vi "FTT Sreen.vi"(8 "error in (no error)":errorcluster caption="错误输入（无错误）", 11 "Main":T2={"Tite"="", "Base path"=path "", "Table"=[], "Stations"=[], "Shield Array"=[], "UPHs"=[], "VISA"={"VISA"="", "baud rate"=9600, "data bits"=8, "parity"=enum."None", "stop bits"=10, "flow control"=0}, "Path"={"roof"=path "", "Config"=path "", "Png"=path ""}, "Ctr"={"DB Dispaly"=refnum, "Error Table"=refnum, "Display"=refnum, "Login"=refnum, "Exit"=refnum, "FTT_Submit"=refnum}, "Login"={"User"="", "Grade"=""}, "information"={"cause"="", "Type"=enum."Inform", "code"=0, "Suroce"="", "Status"=FALSE}, "Local DB"={"Connstr"="", "Database"={"Constr"={"Driver"="", "Server"="", "User"="", "Pwd"="", "Database"=""}, "conn ref"=refnum, "State"=FALSE}}, "Remote DB"={"Connstr"="", "Database"={"Constr"={"Driver"="", "Server"="", "User"="", "Pwd"="", "Database"=""}, "conn ref"=refnum, "State"=FALSE}}, "FTT TV"="", "ExchangeTime"=0, "NVH"="", "EOL Path"=path ""} {"VISA"."flow control" items=["None", "XON/XOFF", "RTS/CTS", "XON/XOFF & RTS/CTS", "DTR/DSR", "XON/XOFF & DTR/DSR"]; "VISA"."stop bits" items=["1.0"=10, "1.5"=15, "2.0"=20]}) -> (0 "error out":errorcluster)   [LabVIEW 2014]
uses:
  Type'def/CN Product1_5 Ctr.ctl
  Type'def/CN Product1_4 Ctr.ctl
  Type'def/CN Product Ctr.ctl
  Type'def/Tab.ctl
  Type'def/MainCtr.ctl
  Type'def/UPH Config.ctl
  SubVI's/VISA/Ctr/VISA Ctr.ctl
  Type'def/Main Ctr Ref.ctl
  Type'def/User Login.ctl
  SubVI's/Database/Ctr/Conneect State.ctl
  SubVI's/Database/Ctr/Constr.ctl
  <vilib>/addons/database/Connection.llb/Conn ObjectReference.ctl
  Type'def/CN image Ctr.ctl
  <vilib>/picture/picture.llb/imagedata.ctl
  Type'def/CN Config Ctr.ctl
  <vilib>/addons/database/NI_Database_API.lvlib
panel:
  out "Tab":T1(array[ring])
  out "size(s)":i32
  out "Value":string
  out "Repaired":string
  out "Slash 04":string
  out "End?":bool
  out "Show Tab":T10
  out "Tab CN":enum32{"1/2", "1/3", "1/4", "1/5", "2/5", "3/5"}(tab)
  out "CN image2/2":T11
  out "CN image1/2":T11
  out "CN image3/3":T11
  out "CN image2/3":T11
  out "CN image1/3":T11
  out "CN image4/4":T12
  out "CN image3/4":T12
  out "CN image2/4":T12
  out "CN image1/4":T12
  out "CN image5/5":T13
  out "CN image4/5":T13
  out "CN image3/5":T13
  out "CN image2/5":T13
  out "CN image1/5":T13
  out "CN image5/6":T13
  out "CN image4/6":T13
  out "CN image3/6":T13
  out "CN image2/6":T13
  out "CN image1/6":T13
  out "CN image5/7":T13
  out "CN image4/7":T13
  out "CN image3/7":T13
  out "CN image2/7":T13
  out "CN image1/7":T13
  out "Roof Picture":picture
  out "Vehicle Picture":picture
  out "Line status":string
  out "UPH status":string
  out "Rollo Color status":string
  out "Model":string
  out "Slash 03":string
  out "Slash 01":string
  out "Slash 02":string
  out "FTT Rate":string
  out "Reject":string
  out "Target(%)":string
  out "Target now":string
  out "FTT":string
  out "Actual":string
  out "Plan":string
  out "Repaired and Reject Title":string
  out "Target and Actual Title":string
  out "FTT and FTT Rate Title":string
  out "Plan and Rate Title":string
  out "Error Info 3":string
  out "Error Info 2":string
  out "Error Info":string
  out "Error BG":u32(colorbox)
  out "Time":string
  out "Date":string
  out "Title":string
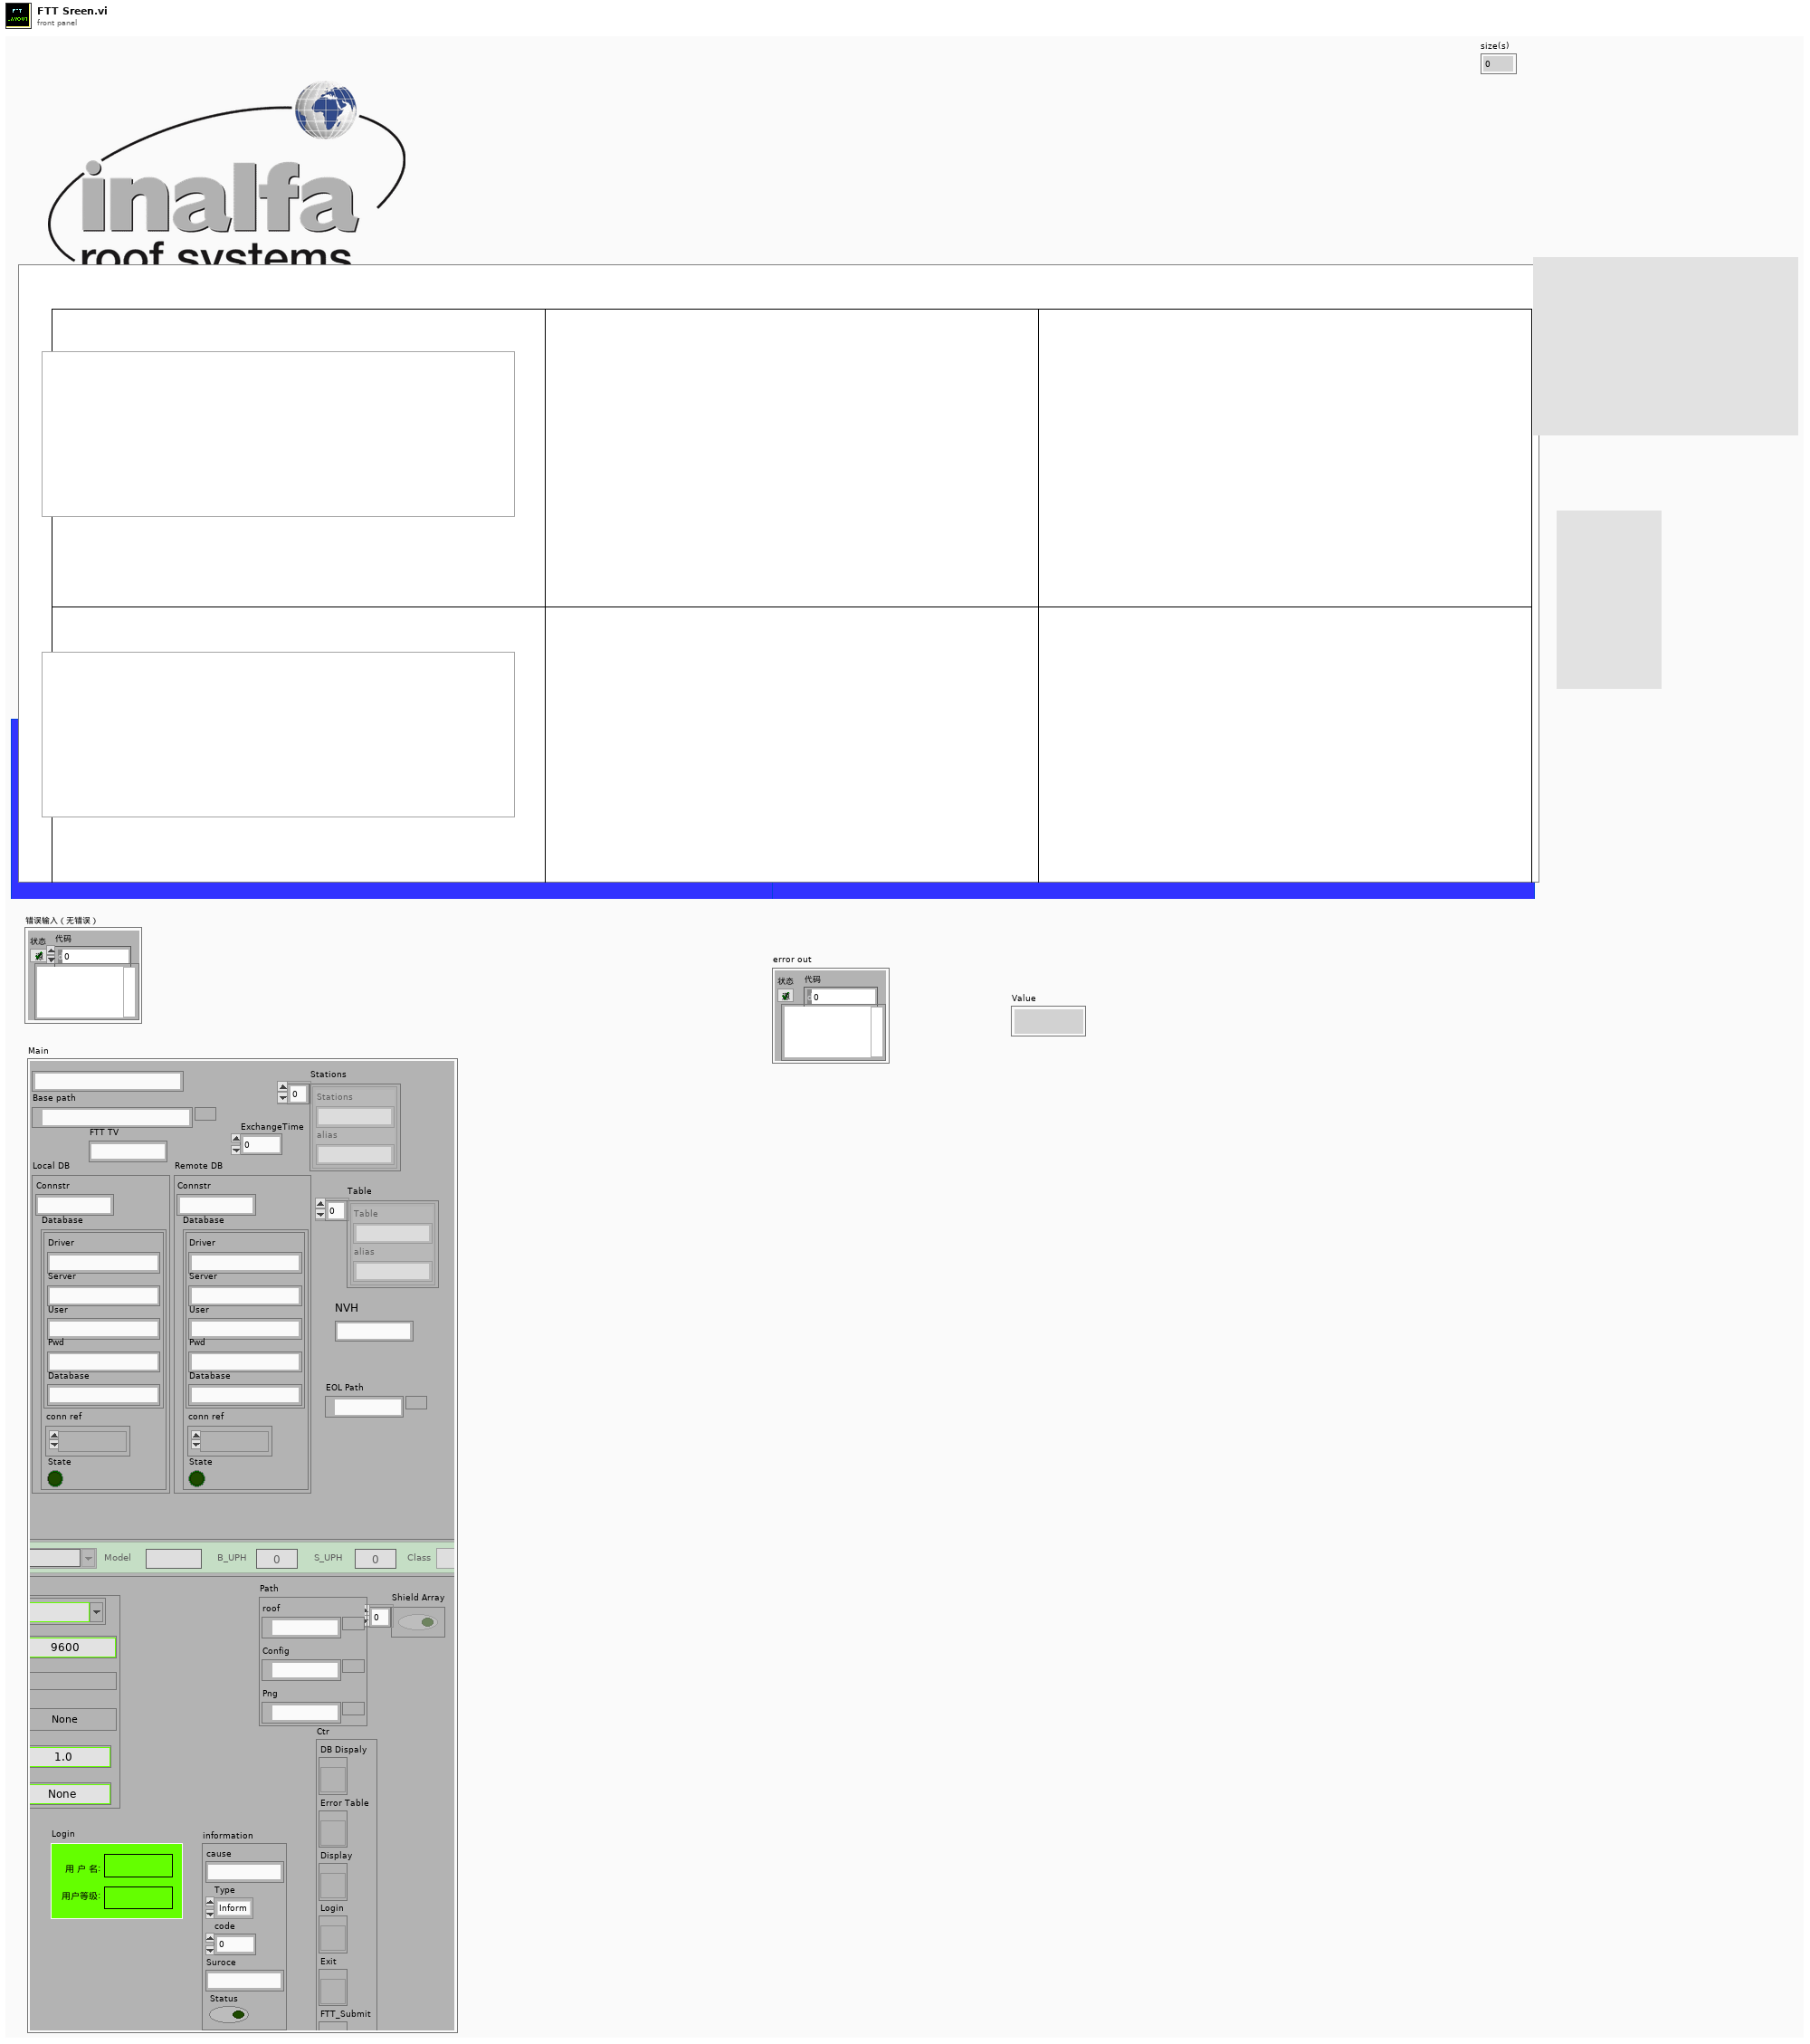
[diagram p1: front panel]
types:
  T1 = enum32{"1/2", "1/3", "1/4", "1/5", "2/5", "3/5"}[]
  T2 = typedef "MainCtr.ctl" = cluster{"Tite":string, "Base path":path, "Table":cluster{"Table":string, "alias":string}[], "Stations":cluster{"Stations":string, "alias":string}[], "Shield Array":bool[], "UPHs":T3[], "VISA":T4, "Path":cluster{"roof":path, "Config":path, "Png":path}, "Ctr":T5, "Login":T6, "information":cluster{"cause":string, "Type":enum16{"Inform", "Warning", "Alarm"}, "code":i32, "Suroce":string, "Status":bool}, "Local DB":cluster{"Connstr":string, "Database":T7}, "Remote DB":cluster{"Connstr":string, "Database":T7}, "FTT TV":string, "ExchangeTime":i32, "NVH":string, "EOL Path":path}
  T3 = typedef "UPH Config.ctl" = cluster{"Line_No":string, "Model":string, "B_UPH ":i16, "S_UPH  ":i16, "Class":enum16{"Big", "Small"}}
  T4 = typedef "VISA Ctr.ctl" = cluster{"VISA":refnum<visa-resource-name>, "baud rate":u32, "data bits":u16, "parity":enum16{"None", "Odd", "Even", "Mark", "Space"}, "stop bits":u16, "flow control":u16}
  T5 = typedef "Main Ctr Ref.ctl" = cluster{"DB Dispaly":refnum<vi>, "Error Table":refnum<vi>, "Display":refnum<vi>, "Login":refnum<vi>, "Exit":refnum<vi>, "FTT_Submit":refnum<vi>}
  T6 = typedef "User Login.ctl" = cluster{"User":string, "Grade":string}
  T7 = typedef "Conneect State.ctl" = cluster{"Constr":T8, "conn ref":T9, "State":bool}
  T8 = typedef "Constr.ctl" = cluster{"Driver":string, "Server":string, "User":string, "Pwd":string, "Database":string}
  T9 = typedef "NI_Database_API.lvlib/Conn ObjectReference.ctl" = refnum<k1>
  T10 = typedef "Tab.ctl" = enum32{"Customer and Shift Info", "Manufacture Info", "Device error info"}
  T11 = typedef "CN Product Ctr.ctl" = cluster{"2D Picture 3":picture, "Model":string, "Brand":string}
  T12 = typedef "CN Product1_4 Ctr.ctl" = cluster{"2D Picture 3":picture, "Model":string, "Brand":string}
  T13 = typedef "CN Product1_5 Ctr.ctl" = cluster{"2D Picture 3":picture, "Model":string, "Brand":string}
  T14 = typedef "imagedata.ctl" = cluster{"image type":i32, "image depth":i32, "image":u8[], "mask":u8[], "colors":u32[], "Rectangle":cluster{"left":i16, "top":i16, "right":i16, "bottom":i16}}
  T15 = cluster{"FTTColor":cluster{"Low":u32, "Middle":u32, "High":u32}, "TargetColor":cluster{"Low":u32, "Middle":u32, "High":u32}}
  T16 = cluster{"FTTRate":cluster{"Low":u32, "High":u32}, "TargetRate":cluster{"Low":u32, "High":u32}}
  T17 = typedef "CN image Ctr.ctl" = cluster{"Images":T14[], "filenames":string[], "Fit Zoom":dbl[], "CN Config":T18[], "CN Enable":T18[], "image Enable":T14[], "CN Ref Enable":refnum<vi>[], "Tab ":enum32{"1/2", "1/3", "1/4", "1/5", "2/5", "3/5"}[], "Pic Enable":refnum<vi>[]}
  T18 = typedef "CN Config Ctr.ctl" = cluster{"Model":string, "Pic_Name":string, "CarName":string, "En/Disable":bool}
  T19 = cluster{"Path":cluster{"roof":path, "Config":path, "Png":path}, "Exit":refnum<vi>, "Show Tab":refnum<vi>, "Target(%)":refnum<vi>, "Repaired":refnum<vi>, "Reject":refnum<vi>, "FTT":refnum<vi>, "FTT Rate":refnum<vi>, "Line status":refnum<vi>, "Vehicle Picture":refnum<vi>, "Roof Picture":refnum<vi>, "Time":refnum<vi>, "Date":refnum<vi>, "Title":refnum<vi>, "Error Info":refnum<vi>, "UPH status":refnum<vi>, "Rollo Color status":refnum<vi>, "Plan":refnum<vi>, "Actual":refnum<vi>, "Repaired":refnum<vi>, "Target now":refnum<vi>, "Range":cluster{"FTTRate":cluster{"Low":u32, "High":u32}, "TargetRate":cluster{"Low":u32, "High":u32}}, "Color":cluster{"FTTColor":cluster{"Low":u32, "Middle":u32, "High":u32}, "TargetColor":cluster{"Low":u32, "Middle":u32, "High":u32}}, "Ctr Color":cluster{"Label":string, "Color":u32}[], "CN Ctr Ref":refnum<vi>[], "CN image":T17, "Tab CN":refnum<vi>}
  T20 = cluster{"seconds":dbl, "Pages":i32, "element":enum32{"1/2", "1/3", "1/4", "1/5", "2/5", "3/5"}}
  T21 = typedef "Main FTT.ctl" = cluster{"Line_Name":string, "Model":string, "Line_State":string, "Color":string, "UPH":string, "Plan":string, "Target Rate":string, "Target":string, "Actual":string, "FTT":string, "FTT Rate":string, "Repaired":string, "Reject":string}
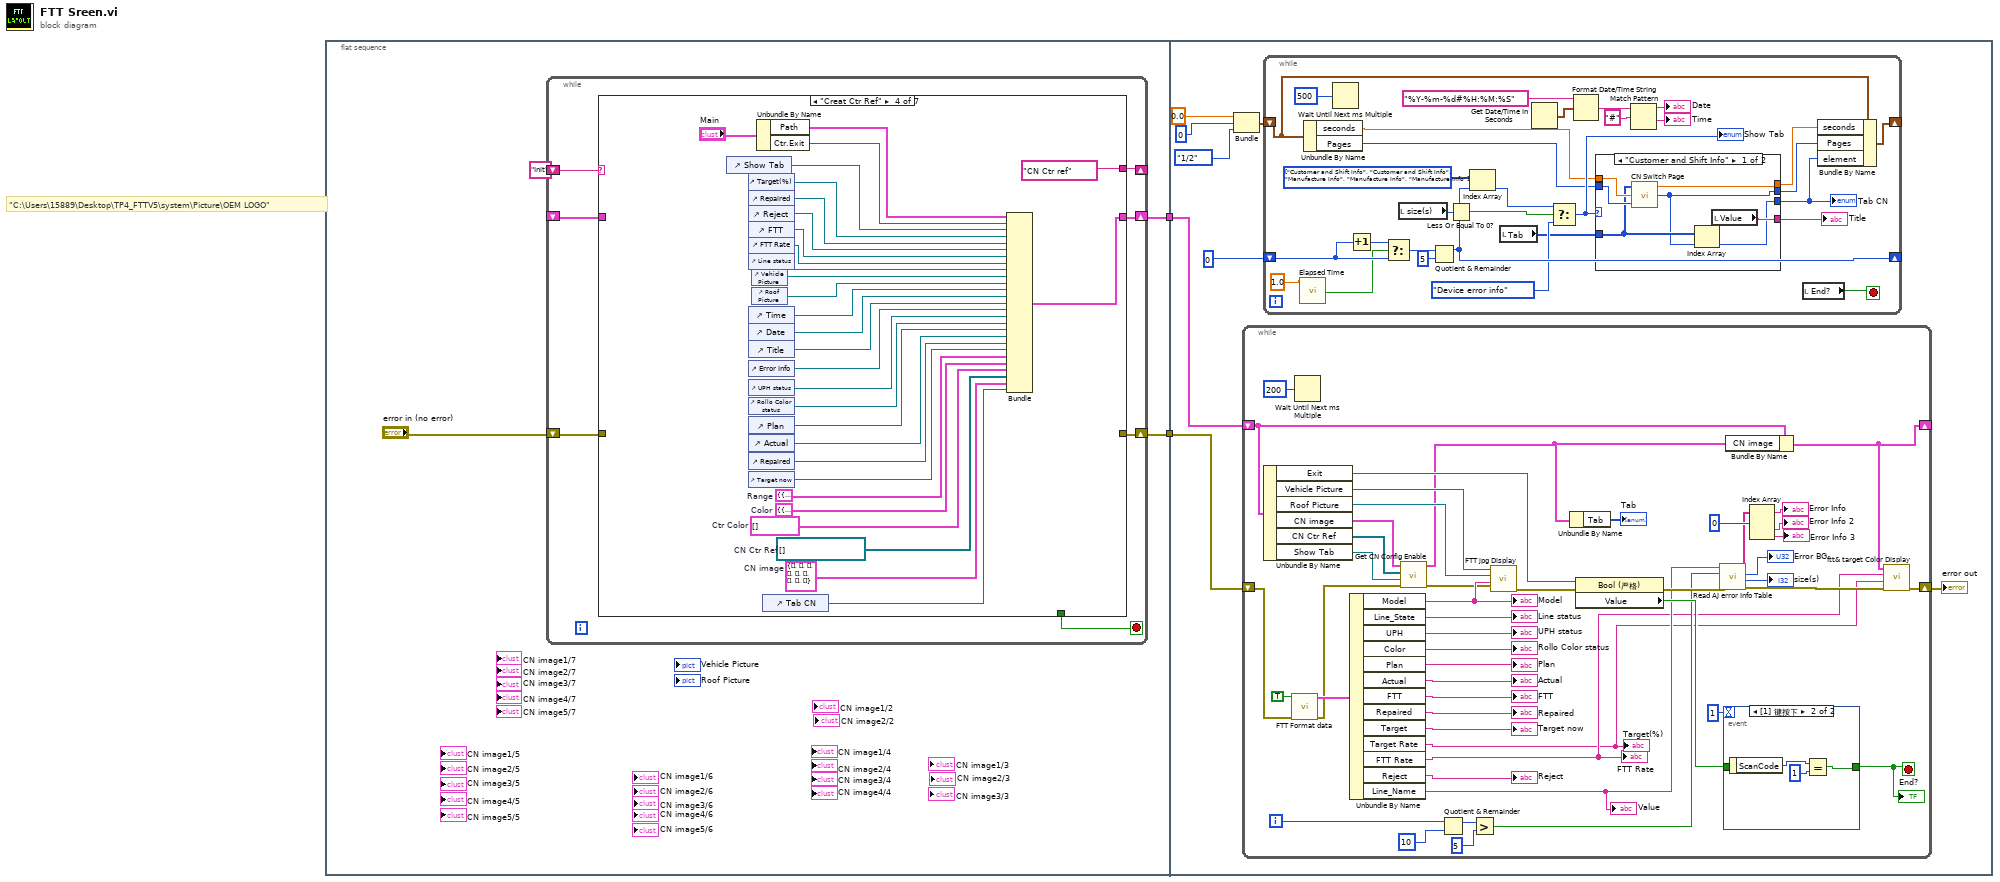
[diagram p0: block diagram]
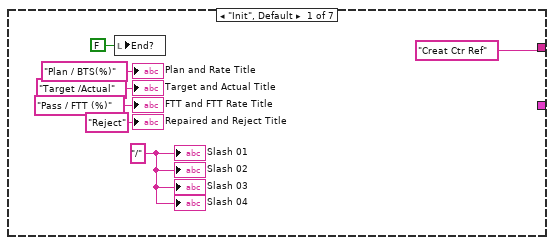
[diagram p2: hidden frame]
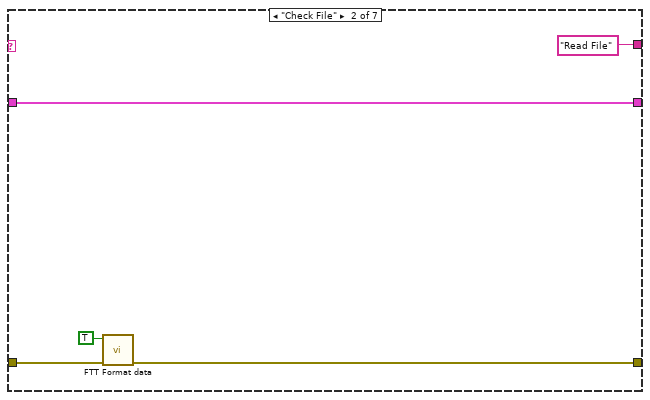
[diagram p3: hidden frame]
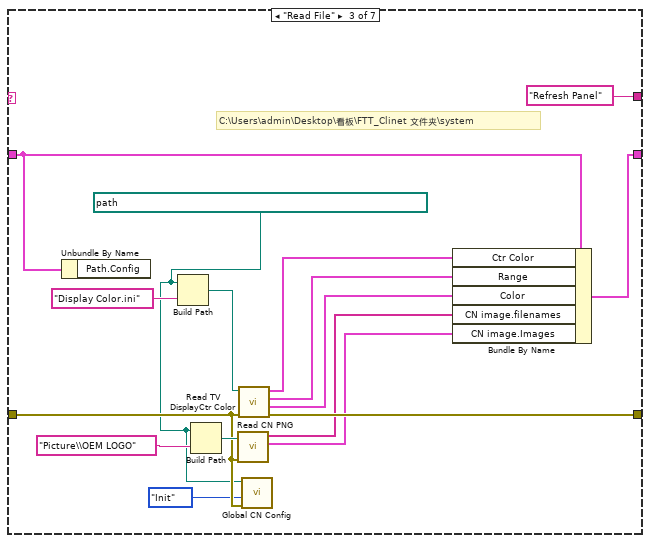
[diagram p4: hidden frame]
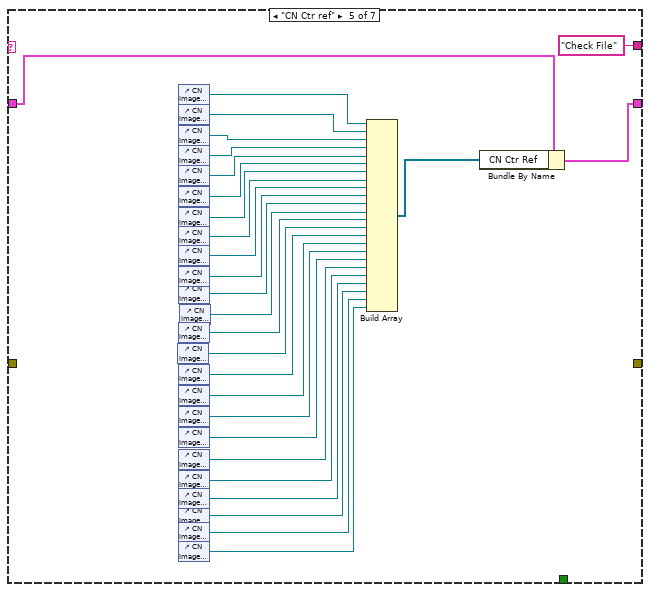
[diagram p5: hidden frame]
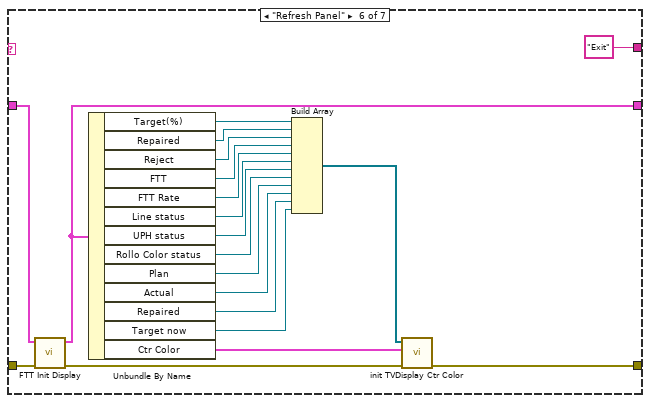
[diagram p6: hidden frame]
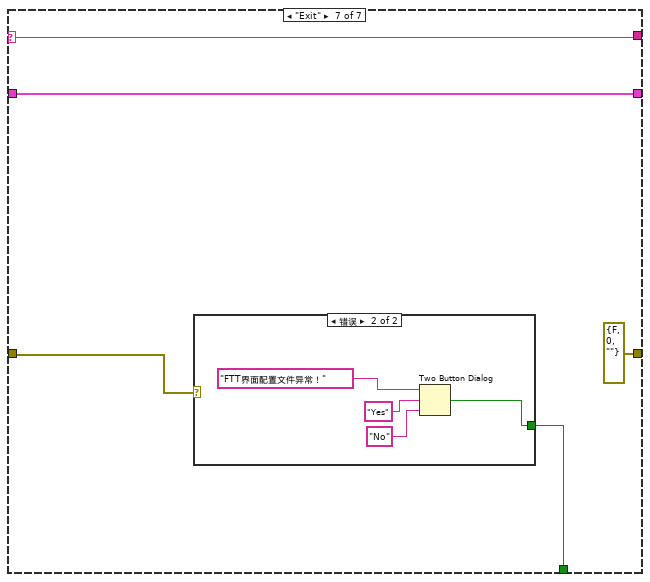
[diagram p7: hidden frame]
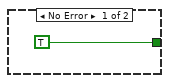
[diagram p8: hidden frame]
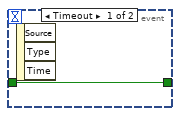
[diagram p9: hidden frame]
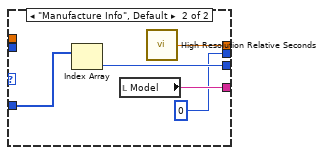
[diagram p10: hidden frame]
diagram:
  # "\"C:\\Users\\15889\\Desktop\\TP4_FTTV5\\system\\Picture\\OEM LOGO\""
  n1 = flat-sequence {
    tunnel: [w4] -> w2
    tunnel: [w3] -> w1
    tunnel: w2 -> [w136]
    tunnel: w1 -> [w137]
    frame #0 {
      n2 = while {
        shift-right: [w12] -> _
        shift-left: "Init" -> [w13]
        shift-right: [w10] -> w3
        shift-left: _ -> [w9]
        shift-right: [w7] -> w4
        shift-left: "error in (no error)" -> [w8]
        stop <- w11 stop-if-true
        n3 = case shown="\"Creat Ctr Ref\"" w13 {
          selector: w13 -> [_ _ _ _ _ _ w123]
          tunnel: ["Creat Ctr Ref" "Read File" "Refresh Panel" "CN Ctr ref" "Check File" "Exit" w123] -> w12
          tunnel: [_ _ _ _ _ _ w120] -> w11
          tunnel: [_ w24 w36 w59 w98 w100 w124] -> w10
          tunnel: w9 -> [_ w24 w37 _ w99 w101 w124]
          tunnel: w8 -> [_ w23 w28 _ _ w118 w121]
          tunnel: [_ w22 w38 _ _ w102 errorcluster {"status"=FALSE, "code"=0, "source"=""} ("error out")] -> w7
          frame "Init", Default {
            w16 = "/" ("Slash 01")
            n4 = local write "End?"(FALSE ("End?")) -> ()
            "FTT and FTT Rate Title" <- "Pass / FTT (%)" ("FTT Title")
            "Plan and Rate Title" <- "Plan / BTS(%)" ("Target and Color Title")
            "Target and Actual Title" <- "Target /Actual" ("FTT Title 3")
            "Repaired and Reject Title" <- "Reject" ("FTT Title 4")
            "Slash 02" <- w16
            "Slash 01" <- w16
            "Slash 03" <- w16
            "Slash 04" <- w16
          }
          frame "Check File" {
            n5 = call "FTT Format data.vi"("error in (no error)"=w23, "W/R"=TRUE) -> ("error out"=w22:errorcluster)  [unwired: 7 in, 2 out]
          }
          frame "Read File" {
            w26 = path "C:/Users/admin/Desktop/看板/FTT_Clinet 文件夹/system" ("Path.Config")
            # "C:\\Users\\admin\\Desktop\\看板\\FTT_Clinet 文件夹\\system"
            n6 = Unbundle By Name(w37) -> ()  [unwired: 1 out]
            n7 = Build Path(base path=w26, name or relative path="Display Color.ini") -> (appended path=w39:path)
            n8 = Build Path(base path=w26, name or relative path="Picture\\OEM LOGO") -> (appended path=w32:path)
            n9 = call "Read CN PNG.vi"("error in (no error)"=w28, "floder Path"=w32) -> ("Images"=w29:T14[], "filenames"=w30:string[])  [unwired: 7 in, 1 out]
            n10 = call "Read TV DisplayCtr Color.vi"("error in (no error)"=w28, "Path"=w39) -> ("error out"=w38:errorcluster, "Color"=w33:T15, "Range"=w34:T16, "Array"=w35:cluster{"Label":string, "Color":u32}[])  [unwired: 6 in]
            n11 = call "Global CN Config.vi"("error in (no error)"=w28, "Mode"=enum16{"Init", "Read", "Write"}."Init", "Path"=w26) -> ()  [unwired: 7 in, 2 out]
            n12 = Bundle By Name(cluster=w37, "Ctr Color"=w35, "Range"=w34, "Color"=w33, "CN image.filenames"=w30, "CN image.Images"=w29) -> (w36:T19)
          }
          frame "Creat Ctr Ref" {
            w43 = T17 {"Images"=[], "filenames"=[], "Fit Zoom"=[], "CN Config"=[], "CN Enable"=[], "image Enable"=[], "CN Ref Enable"=[], "Tab "=[], "Pic Enable"=[]}  # CN image
            w44 = refnum<vi>[] []  # CN Ctr Ref
            w47 = cluster{"Label":string, "Color":u32}[] []  # Ctr Color
            w48 = T15 {"FTTColor"={"Low"=0, "Middle"=0, "High"=0}, "TargetColor"={"Low"=0, "Middle"=0, "High"=0}}  # Color
            w49 = T16 {"FTTRate"={"Low"=0, "High"=0}, "TargetRate"={"Low"=0, "High"=0}}  # Range
            n13 = control-ref of="Show Tab"() -> (w71:refnum<vi>)
            n14 = control-ref of="Target(%)"() -> (w70:refnum<vi>)
            n15 = control-ref of="Repaired"() -> (w69:refnum<vi>)
            n16 = control-ref of="Reject"() -> (w68:refnum<vi>)
            n17 = control-ref of="FTT"() -> (w67:refnum<vi>)
            n18 = control-ref of="FTT Rate"() -> (w66:refnum<vi>)
            n19 = control-ref of="Line status"() -> (w65:refnum<vi>)
            n20 = control-ref of="Time"() -> (w62:refnum<vi>)
            n21 = control-ref of="Date"() -> (w61:refnum<vi>)
            n22 = control-ref of="Title"() -> (w60:refnum<vi>)
            n23 = control-ref of="Error Info"() -> (w56:refnum<vi>)
            n24 = control-ref of="UPH status"() -> (w55:refnum<vi>)
            n25 = control-ref of="Rollo Color status"() -> (w54:refnum<vi>)
            n26 = control-ref of="Plan"() -> (w53:refnum<vi>)
            n27 = control-ref of="Actual"() -> (w52:refnum<vi>)
            n28 = control-ref of="Repaired"() -> (w51:refnum<vi>)
            n29 = control-ref of="Target now"() -> (w50:refnum<vi>)
            n30 = control-ref of="Vehicle Picture"() -> (w64:refnum<vi>)
            n31 = control-ref of="Roof Picture"() -> (w63:refnum<vi>)
            n32 = Unbundle By Name("Main") -> ("Path"=w45:cluster{"roof":path, "Config":path, "Png":path}, "Ctr.Exit"=w57:refnum<vi>)
            n33 = control-ref of="Tab CN"() -> (w42:refnum<vi>)
            n34 = Bundle("Path"=w45, "Exit"=w57, "Show Tab"=w71, "Target(%)"=w70, "Repaired"=w69, "Reject"=w68, "FTT"=w67, "FTT Rate"=w66, "Line status"=w65, "Vehicle Picture"=w64, "Roof Picture"=w63, "Time"=w62, "Date"=w61, "Title"=w60, "Error Info"=w56, "UPH status"=w55, "Rollo Color status"=w54, "Plan"=w53, "Actual"=w52, "Repaired"=w51, "Target now"=w50, "Range"=w49, "Color"=w48, "Ctr Color"=w47, "CN Ctr Ref"=w44, "CN image"=w43, "Tab CN"=w42) -> (w59:T19)  [unwired: 1 in]
          }
          frame "CN Ctr ref" {
            n35 = control-ref of="CN image5/5"() -> (w84:refnum<vi>)
            n36 = control-ref of="CN image1/2"() -> (w97:refnum<vi>)
            n37 = control-ref of="CN image2/2"() -> (w96:refnum<vi>)
            n38 = control-ref of="CN image1/3"() -> (w95:refnum<vi>)
            n39 = control-ref of="CN image2/3"() -> (w94:refnum<vi>)
            n40 = control-ref of="CN image3/3"() -> (w93:refnum<vi>)
            n41 = control-ref of="CN image1/4"() -> (w92:refnum<vi>)
            n42 = control-ref of="CN image2/4"() -> (w91:refnum<vi>)
            n43 = control-ref of="CN image3/4"() -> (w90:refnum<vi>)
            n44 = control-ref of="CN image4/4"() -> (w89:refnum<vi>)
            n45 = control-ref of="CN image1/5"() -> (w88:refnum<vi>)
            n46 = control-ref of="CN image2/5"() -> (w87:refnum<vi>)
            n47 = control-ref of="CN image4/5"() -> (w85:refnum<vi>)
            n48 = control-ref of="CN image1/6"() -> (w83:refnum<vi>)
            n49 = control-ref of="CN image2/6"() -> (w82:refnum<vi>)
            n50 = control-ref of="CN image3/6"() -> (w81:refnum<vi>)
            n51 = control-ref of="CN image4/6"() -> (w80:refnum<vi>)
            n52 = control-ref of="CN image5/6"() -> (w79:refnum<vi>)
            n53 = control-ref of="CN image1/7"() -> (w78:refnum<vi>)
            n54 = control-ref of="CN image2/7"() -> (w77:refnum<vi>)
            n55 = control-ref of="CN image3/7"() -> (w76:refnum<vi>)
            n56 = control-ref of="CN image4/7"() -> (w75:refnum<vi>)
            n57 = control-ref of="CN image5/7"() -> (w74:refnum<vi>)
            n58 = control-ref of="CN image3/5"() -> (w86:refnum<vi>)
            n59 = Build Array(w97, w96, w95, w94, w93, w92, w91, w90, w89, w88, w87, w86, w85, w84, w83, w82, w81, w80, w79, w78, w77, w76, w75, w74) -> (w73:refnum<vi>[])
            n60 = Bundle By Name(cluster=w99, "CN Ctr Ref"=w73) -> (w98:T19)
          }
          frame "Refresh Panel" {
            n61 = call "FTT Init Display.vi"("error in (no error)"=w118, "Cluster 2"=w101) -> ("error out"=w105:errorcluster, "Cluster out"=w100:T19)  [unwired: 8 in]
            n62 = Unbundle By Name(w100) -> ("Target(%)"=w117:refnum<vi>, "Repaired"=w116:refnum<vi>, "Reject"=w115:refnum<vi>, "FTT"=w114:refnum<vi>, "FTT Rate"=w113:refnum<vi>, "Line status"=w112:refnum<vi>, "UPH status"=w111:refnum<vi>, "Rollo Color status"=w110:refnum<vi>, "Plan"=w109:refnum<vi>, "Actual"=w108:refnum<vi>, "Repaired"=w107:refnum<vi>, "Target now"=w106:refnum<vi>, "Ctr Color"=w103:cluster{"Label":string, "Color":u32}[])
            n63 = Build Array(w117, w116, w115, w114, w113, w112, w111, w110, w109, w108, w107, w106) -> (w104:refnum<vi>[])
            n64 = call "init TVDisplay Ctr Color.vi"("error in (no error)"=w105, "Ctr Color"=w103, "appended array"=w104) -> ("error out"=w102:errorcluster)  [unwired: 8 in]
          }
          frame "Exit" {
            n65 = case shown="错误" w121 {
              tunnel: [TRUE w126] -> w120
              frame No Error {
              }
              frame Error {
                n66 = Two Button Dialog(message="FTT界面配置文件异常！" ("消息"), 1:"No" ("F按钮名称（“取消”）"), 2:"Yes" ("T按钮名称（“确定”）")) -> (T button?=w126:bool)
              }
            }
          }
        }
      }
    }
    frame #1 {
      n67 = Bundle("seconds"=0.0, "Pages"=0, "element"=enum32{"1/2", "1/3", "1/4", "1/5", "2/5", "3/5"}."1/2") -> (w130:T20)  [unwired: 1 in]
      n68 = while {
        shift-right: [w149] -> w135
        shift-left: w136 -> [w177]
        shift-right: [w140] -> _
        shift-left: w137 -> [w143]
        i -> [w163]
        stop <- w165 stop-if-true
        n69 = Unbundle By Name(w143) -> ("Exit"=w167:refnum<vi>, "Vehicle Picture"=w184:refnum<vi>, "Roof Picture"=w183:refnum<vi>, "CN image"=w146:T17, "CN Ctr Ref"=w142:refnum<vi>[], "Show Tab"=w141:refnum<vi>)
        n70 = call "FTT Format data.vi"("error in (no error)"=w177, "W/R"=TRUE) -> ("error out"=w145:errorcluster, "Display"=w182:T21)  [unwired: 7 in, 1 out]
        n71 = Wait Until Next ms Multiple(millisecond multiple=u32 200) -> ()  [unwired: 1 out]
        n72 = Unbundle By Name(w182) -> ("Model"=w180:string, "Line_State"=→"Line status":string, "UPH"=→"UPH status":string, "Color"=→"Rollo Color status":string, "Plan"=→"Plan":string, "Actual"=→"Actual":string, "FTT"=→"FTT":string, "Repaired"=→"Repaired":string, "Target"=→"Target now":string, "Target Rate"=w147:string, "FTT Rate"=w148:string, "Reject"=→"Reject":string, "Line_Name"=w151:string)
        "Model" <- w180
        "Target(%)" <- w147
        "FTT Rate" <- w148
        "Value" <- w151
        n73 = call "Get CN Config Enable.vi"("error in (no error)"=w145, "Show Tab"=w141, "CN Pic Ref"=w142, "CN image"=w146) -> ("error out"=w144:errorcluster, "CN image out"=w139:T17)  [unwired: 6 in]
        n74 = Quotient & Remainder(x=w163, y=10) -> (x-y*floor(x/y)=w161:i32)  [unwired: 1 out]
        n75 = Greater?(x=w161, y=5) -> (0:w159:bool)
        n76 = call "FTT jpg Display.vi"("error in (no error)"=w144, "Model"=w180, "Roof Picture"=w183, "Vehicle Picture"=w184) -> ("错误输出"=w168:errorcluster)  [unwired: 7 in]
        n77 = Unbundle By Name(w139) -> ("Tab"=→"Tab":T1)
        n78 = property class="Bool (严格)"(reference=w167, error in=w168) -> (error out=w164:errorcluster, "Value"=w166:bool)  [unwired: 1 out]
        n79 = call "Read AJ error Info Table.vi"("error in (no error)"=w164, "s"=w159, "Linename"=w151) -> ("error IO"=w150:errorcluster, "size(s)"=→"size(s)":i32, "Error BG"=→"Error BG":u32, "Array"=w152:string[])  [unwired: 5 in]
        n80 = event shown="[1] 键按下" {
          selector: _ -> [_ _]
          dyn-events: _ -> [_ _]
          timeout: 1 -> [_ _]
          tunnel: [w186 w187] -> w165
          tunnel: w166 -> [w186 _]
          event Timeout {
            n81 = event-data() -> ()  [unwired: 1 in, 3 out]
          }
          event Key Down {
            n82 = event-data() -> ("ScanCode"=w189:i16)  [unwired: 1 in]
            n83 = Equal?(x=w189, y=i16 1) -> (x = y?=w187:bool)
          }
        }
        "End?" <- w165
        n84 = Bundle By Name(cluster=w143, "CN image"=w139) -> (w140:T19)
        n85 = Index Array(array=w152, index #1=0 ("index")) -> (element #1=→"Error Info":string, element #2=→"Error Info 2":string, element #3=→"Error Info 3":string)  [unwired: 2 in]
        n86 = call "ftt& target Color Display.vi"("error in (no error)"=w150, "Tatget"=w147, "ftt"=w148, "Cluster"=w140) -> ("error out"=w149:errorcluster)  [unwired: 7 in]
      }
      "error out" <- w135
      n87 = while {
        shift-right: [w208] -> _
        shift-left: u64 0 -> [w217]
        shift-right: [w195] -> _
        shift-left: w130 -> [w196]
        stop <- w204 stop-if-true
        w215 = T10[] [enum."Customer and Shift Info", enum."Customer and Shift Info", enum."Manufacture Info", enum."Manufacture Info", enum."Manufacture Info"] items=["Customer and Shift Info", "Manufacture Info", "Device error info"]
        n88 = call "Elapsed Time"("Time Target (s)"=1.0) -> ("Time has Elapsed"=w203:bool)  [unwired: 11 in, 7 out]
        n89 = Unbundle By Name(w196) -> ("seconds"=w191:dbl, "Pages"=w190:i32)
        n90 = Wait Until Next ms Multiple(millisecond multiple=u32 500) -> ()  [unwired: 1 out]
        n91 = Increment(x=w217) -> (x+1=w216:u64)
        n92 = Select(t=w216, s=w203, f=w217) -> (s? t:f=w210:u64)
        n93 = local read "size(s)"() -> (w199:i32)
        n94 = Quotient & Remainder(x=w210, y=u64 5) -> (x-y*floor(x/y)=w208:u64)  [unwired: 1 out]
        n95 = Less Or Equal To 0?(x=w199) -> (x <= 0?=w198:bool)
        n96 = Index Array(array=w215, index=w208) -> (element=w201:T10)
        n97 = local read "Tab"() -> (w197:T1)
        n98 = Get Date/Time In Seconds() -> (seconds since 1Jan1904=w211:timestamp)
        n99 = Select(t=w201, s=w198, f=Tab."Device error info" ("element")) -> (s? t:f=w200:T10)
        "Show Tab" <- w200
        n100 = Format Date/Time String(time format string (%c)="%Y-%m-%d#%H:%M:%S", seconds (now)=w211) -> (date/time string=w212:string)  [unwired: 1 in]
        n101 = case shown="\"Customer and Shift Info\"" w200 {
          tunnel: [w226 w231] -> w207
          tunnel: w197 -> [w222 w230]
          tunnel: [w220 w229] -> w192
          tunnel: [w223 w228] -> w194
          tunnel: [w221 0] -> w193
          tunnel: w191 -> [w225 _]
          tunnel: w190 -> [w224 _]
          frame "Customer and Shift Info" {
            n102 = call "CN Switch Page.vi"("Page"=w224, "Scond"=w225, "Tab"=w222) -> ("Page"=w221:i32, "scond"=w223:dbl)  [unwired: 1 out]
            n103 = Index Array(array=w222, index=w221) -> (element=w220:enum32{"1/2", "1/3", "1/4", "1/5", "2/5", "3/5"})
            n104 = local read "Value"() -> (w226:string)
          }
          frame "Manufacture Info", Default {
            n105 = Index Array(array=w230) -> (element=w229:enum32{"1/2", "1/3", "1/4", "1/5", "2/5", "3/5"})  [unwired: 1 in]
            n106 = local read "Model"() -> (w231:string)
            n107 = call <vilib>:"High Resolution Relative Seconds.vi"() -> ("relative seconds"=w228:dbl)
          }
        }
        "Title" <- w207
        "Tab CN" <- w192
        n108 = Match Pattern(string=w212, regular expression="#") -> (before substring=→"Date":string, after substring=→"Time":string)  [unwired: 1 in, 2 out]
        n109 = local read "End?"() -> (w204:bool)
        n110 = Bundle By Name(cluster=w196, "seconds"=w194, "Pages"=w193, "element"=w192) -> (w195:T20)
      }
    }
  }
